vi "Fft-16.vi"() -> ()   [LabVIEW 2014]
uses:
  <vilib>/Platform/TimedLoop/XDataNode/timing_clust.ctl
  <vilib>/Platform/TimedLoop/XDataNode/nitl_modes.ctl
  <vilib>/Platform/TimedLoop/XDataNode/wakeup.ctl
  <vilib>/rvi/Analysis/measure/FFT/simModelSupport/niFPGA FFT Sim Properties.ctl
  <vilib>/rvi/Analysis/measure/FFT/simModelSupport/niFPGA FFT Sim Types.ctl
  <vilib>/rvi/Analysis/measure/FFT/simModelSupport/niFpgaFFTSimArithmeticProperties.ctl
  <vilib>/rvi/Analysis/measure/FFT/simModelSupport/niFpgaFFTSimDfxp.ctl
  <vilib>/fxp/LVFixedPointQuantizationPolicyTypeDef.ctl
  <vilib>/rvi/Emulation/niFpgaSctlEmulationGetInTimedLoop.vi
  <vilib>/rvi/Emulation/niFpgaEmulationReportErrorSimple.vi
  <vilib>/rvi/Emulation/niFpgaGetClockAttributes.vi
  <vilib>/rvi/Emulation/niFpgaCriticalErrorInLSC.vi
  <vilib>/rvi/interface/RandomDataEmulation/niFpgaRandomDataHandleErrors.vi
  <vilib>/rvi/Emulation/niFpgaEmulationIsFPGAContextNoSignature.vi
  <vilib>/rvi/errors/niFpgaSetErrorForExecOnDevCompSimple.vi
  <vilib>/rvi/eio/common/nirviEmuReportErrorAndStop.vi
  <vilib>/rvi/DataTransferAndStorage/Container/Common/niFpgaContainerGetUniqueNameForEmu.vi
  <vilib>/rvi/FIFO/Fifo_Resource/nirvififoEmulationSetSize.vi
  <vilib>/rvi/FIFO/Fifo_Resource/nirviFifoEmulationQueueMgr.vi
  <instcachedir>/0/nirviFifoEmulationQueueMgr_E5CAEC123FF24DC58D834DCA3CDAA9B5.lvgen/nirviFifoEmulationQueueMgr_E5CAEC123FF24DC58D834DCA3CDAA9B5_002.vi
  <vilib>/rvi/FIFO/Fifo_Resource/nirvififoEmulationDetermineInputValidOut.vi
  <vilib>/rvi/FIFO/Fifo_Resource/nirvififoEmulationCreateLock.vi
  <vilib>/rvi/Emulation/niFpgaProcessEmulError.vi
  <vilib>/rvi/FIFO/Fifo_Resource/nirvififoEmulationObtainLock.vi
  <vilib>/rvi/FIFO/Fifo_Resource/nirvififoEmulationReleaseLock.vi
  <vilib>/rvi/occurrence/nirviWaitOnOccurrenceBase.vi
  <vilib>/rvi/errors/nirviReportUnexpectedCaseInternalError.vi
  <vilib>/rvi/errors/nirviReportUnexpectedCaseInternalError (U32).vi
  <vilib>/rvi/Analysis/measure/FFT/simModelSupport/niFpgaFFTSimModelCore.vi
  <vilib>/Utility/error.llb/Clear Errors.vi
  <vilib>/Platform/TimedLoop/XDataNode/XDataNode.xnode
  <vilib>/rvi/DataTransferAndStorage/Container/XNode/niFpgaContainer.xnode
  <vilib>/rvi/interface/RandomDataEmulation/nirviRandomDataFpgaReadWriteTemplate.vi
  <vilib>/rvi/FIFO/Fifo_Resource/nirvififoEmulationWrite.vi
  <vilib>/rvi/Analysis/measure/FFT/XNode/niFpgaFFT.xnode
  <vilib>/rvi/FIFO/Fifo_Resource/nirvififoEmulationRead.vi
  <vilib>/Platform/TimedLoop/XDataNode/XDNodeRunTimeDep.lvlib
panel:
  out "output valid":bool
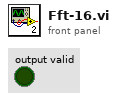
[diagram p1: front panel]
types:
  T1 = typedef "XDNodeRunTimeDep.lvlib/timing_clust.ctl" = cluster{"Expected End [f-1]":u64, "Actual End [f-1]":u64, "Finished Late? [f-1]":bool, "Expected End [i-1]":u64, "Actual End [i-1]":u64, "Finished Late? [i-1]":bool, "Expected Start [i]":u64, "Actual Start [i]":u64, "Expected Start [f]":u64, "Actual Start [f]":u64, "Source Name":string, "Structure Name":string, "Period":i64, "Deadline":i64, "Offset":i64, "Start":i64, "Priority":i32, "Timeout":i32, "Mode":T2, "Wakeup Reason":T3, "Error":errorcluster, "Source Type":string, "Secondary Source Type":string, "Global End Time":u64, "Global Start Time":u64, "Frame Duration":u64, "Iteration Duration":u64, "Assigned CPU":i32, "I/O Scan Engine Mode":u32}
  T2 = typedef "XDNodeRunTimeDep.lvlib/nitl_modes.ctl" = enum32{"No Change", "Process missed periods, maintain original phase", "Discard missed periods, maintain original phase", "Process missed periods, ignore original phase", "Discard missed periods, ignore original phase"}
  T3 = typedef "XDNodeRunTimeDep.lvlib/wakeup.ctl" = enum32{"Normal", "Aborted", "Asynchronous wakeup", "Timing source error", "Timed loop error", "Timeout"}
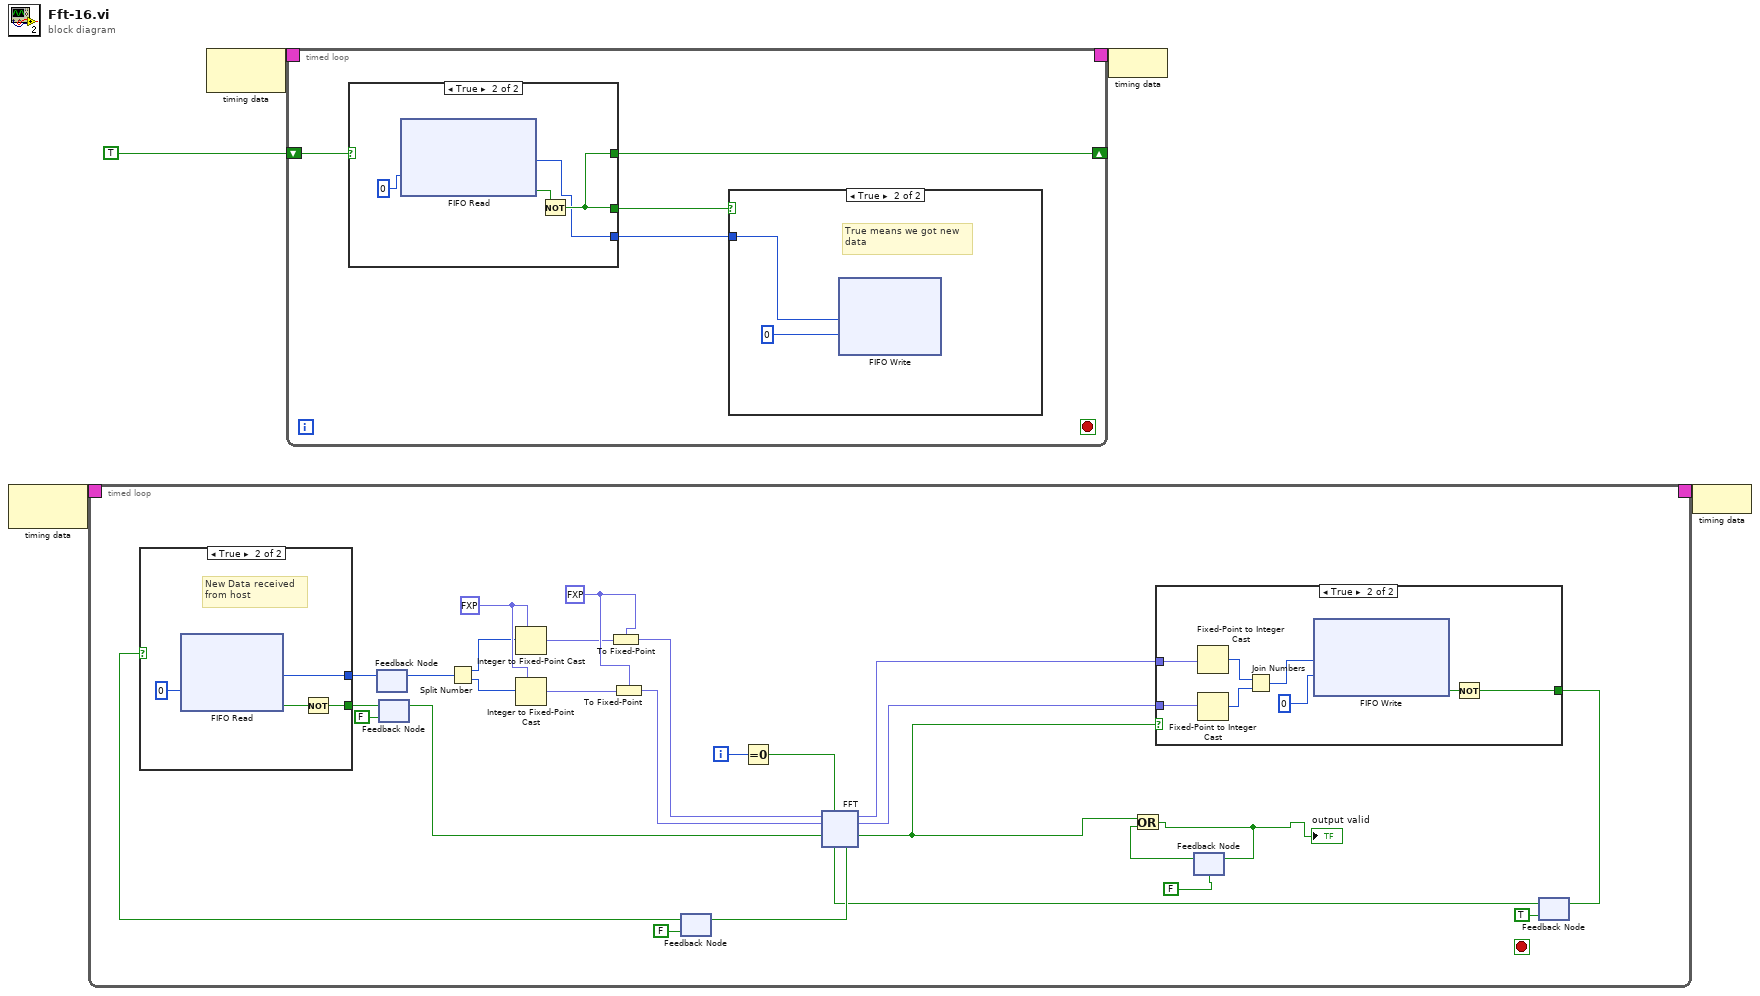
[diagram p0: block diagram]
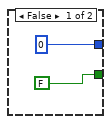
[diagram p2: hidden frame]
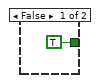
[diagram p3: hidden frame]
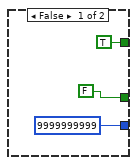
[diagram p5: hidden frame]
diagram:
  n1 = node-c288() -> (w2:T1)  [unwired: 1 in]
  n2 = timed-loop {
    timing: w2 -> [_]
    timing-out: [_] -> w1
    i -> [w21]
    stop <- _ stop-if-true
    w17 = fxp<+/-,24,7> 0.0 ("real data in")
    w20 = fxp<+/-,32,7> 0.0 ("real data in")
    n3 = feedback #1() -> (w12:u64)  [unwired: 1 in]
    n4 = feedback #2(FALSE ("Timed Out?")) -> (w11:bool)
    n5 = Split Number(x=w12) -> (hi(x)=w19:u32, lo(x)=w30:u32)
    n6 = Integer to Fixed-Point Cast(fixed-point type=w20, integer=w19) -> (fixed-point=w14:fxp<+/-,32,7>)
    n7 = Integer to Fixed-Point Cast(fixed-point type=w20, integer=w30) -> (fixed-point=w15:fxp<+/-,32,7>)
    n8 = To Fixed-Point(fixed-point type=w17, number=w14) -> (fixed-point=w16:fxp<+/-,24,7>)
    n9 = To Fixed-Point(fixed-point type=w17, number=w15) -> (fixed-point=w18:fxp<+/-,24,7>)
    n10 = feedback #3(FALSE ("ready for data")) -> (w26:bool)
    n11 = case shown="True" w26 {
      tunnel: [FALSE ("Timed Out?") w38] -> w13
      tunnel: [u64 0 ("Element") w35] -> w29
      frame False {
      }
      frame True {
        # "New Data received \nfrom host"
        n12 = xnode "FIFO Read"("Timeout"=0) -> ("Element"=w35:u64, "Timed Out?"=w36:bool)  [unwired: 1 in, 1 out]
        n13 = Not(x=w36) -> (.not. x?=w38:bool)
      }
    }
    n14 = feedback-in #1(w29) -> ()
    n15 = feedback-in #2(w13) -> ()
    n16 = Equal To 0?(x=w21) -> (x = 0?=w7:bool)
    n17 = feedback #4(FALSE) -> (w23:bool)
    n18 = feedback #5(TRUE ("Timed Out?")) -> (w27:bool)
    n19 = xnode "FFT"("real data in"=w16, "reset"=w7, "imaginary data in"=w18, "input valid"=w11, "ready for output"=w27) -> ("ready for input"=w31:bool, "real data out"=w9:fxp<+/-,32,12>, "imaginary data out"=w8:fxp<+/-,32,12>, "output valid"=w10:bool)  [unwired: 1 out]
    n20 = feedback-in #3(w31) -> ()
    n21 = Or(x=w10, y=w23) -> (x .or. y?=w22:bool)
    "output valid" <- w22
    n22 = case shown="True" w10 {
      tunnel: w9 -> [_ w40]
      tunnel: w8 -> [_ w45]
      tunnel: [TRUE ("Timed Out?") w41] -> w28
      frame False {
      }
      frame True {
        n23 = Fixed-Point to Integer Cast(1:w40) -> (0:w47:i32)
        n24 = Fixed-Point to Integer Cast(1:w45) -> (0:w46:i32)
        n25 = Join Numbers(hi=w47, lo=w46) -> ((hi.lo)=w44:u64)
        n26 = xnode "FIFO Write"("Element"=w44, "Timeout"=0) -> ("Timed Out?"=w42:bool)  [unwired: 1 in, 1 out]
        n27 = Not(x=w42) -> (.not. x?=w41:bool)
      }
    }
    n28 = feedback-in #4(w22) -> ()
    n29 = feedback-in #5(w28) -> ()
  }
  n30 = node-c288() -> (w5:T1)  [unwired: 1 in]
  n31 = timed-loop {
    timing: w5 -> [_]
    timing-out: [_] -> w4
    shift-right: [w77] -> _
    shift-left: TRUE -> [w79]
    stop <- _ stop-if-true
    n32 = case shown="True" w79 {
      tunnel: [TRUE w88] -> w77
      tunnel: [u64 9999999999 ("Element") w85] -> w78
      tunnel: [FALSE w88] -> w76
      frame False {
      }
      frame True {
        n33 = xnode "FIFO Read"("Timeout"=0) -> ("Element"=w85:u64, "Timed Out?"=w86:bool)  [unwired: 1 in, 1 out]
        n34 = Not(x=w86) -> (.not. x?=w88:bool)
      }
    }
    n35 = case shown="True" w76 {
      tunnel: w78 -> [_ w80]
      frame False {
      }
      frame True {
        # "True means we got new\ndata"
        n36 = xnode "FIFO Write"("Element"=w80, "Timeout"=0) -> ()  [unwired: 1 in, 2 out]
      }
    }
  }
  n37 = node-c288(w4) -> ()
  n38 = node-c288(w1) -> ()
